vi "create_cache_directory_if_nonexistent.vi"(8 "error in (no error)":errorcluster, 10 "cache file":path, 11 "exists":bool) -> (0 "error out":errorcluster, 3 "cache file path":path)   [LabVIEW 2016]
uses:
  <userlib>/_OpenG.lib/file/file.llb/Strip Path - Traditional__ogtk.vi
  <userlib>/_OpenG.lib/file/file.llb/Build Path - Traditional__ogtk.vi
panel:
  out "created folders":bool
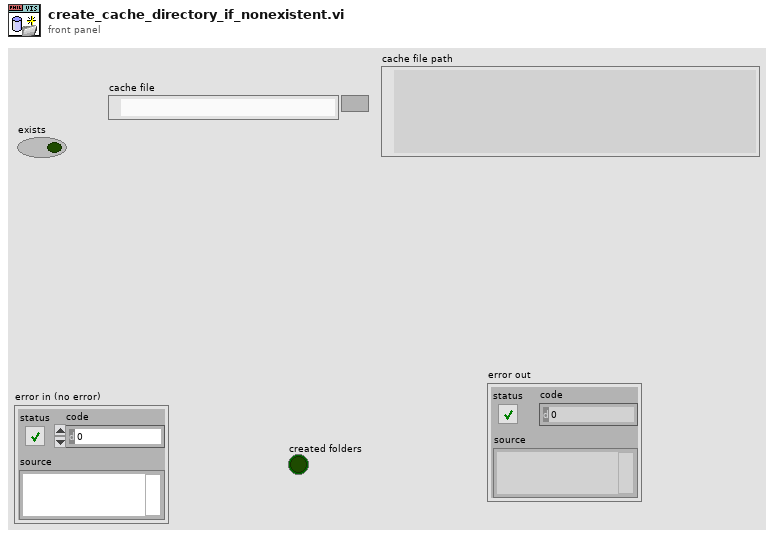
[diagram p1: front panel]
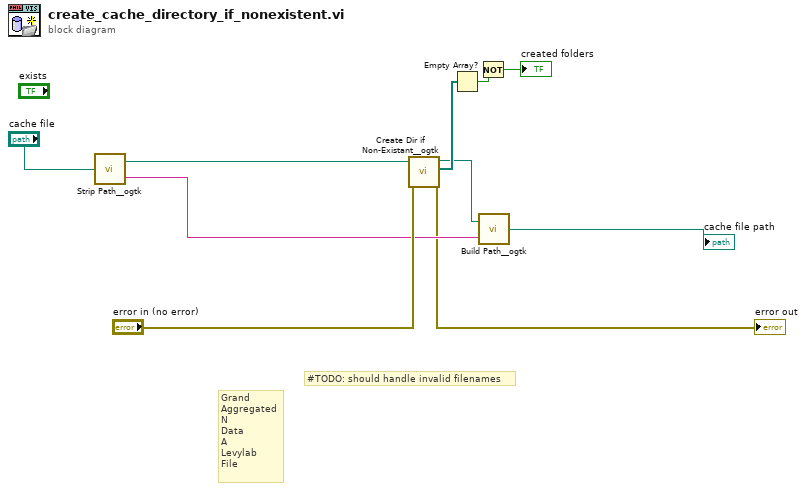
[diagram p0: block diagram]
diagram:
  # "Grand\nAggregated\nN\nData\nA\nLevylab\nFile"
  # "#TODO: should handle invalid filenames"
  n1 = call-poly <userlib>:"Strip Path__ogtk.vi"("path"="cache file") -> ("stripped path"=w4:path, "name"=w3:string)
  n2 = call <userlib>:"Create Dir if Non-Existant__ogtk.vi"("error in (no error)"="error in (no error)", "Directory Path"=w4) -> ("error out"=→"error out":errorcluster, "Created Directories"=w9:path[], "dup Directory Path"=w6:path)  [unwired: 7 in]
  n3 = Empty Array?(array=w9) -> (empty?=w8:bool)
  n4 = Not(x=w8) -> (.not. x?=→"created folders":bool)
  n5 = call-poly <userlib>:"Build Path__ogtk.vi"("name or relative path"=w3, "base path"=w6) -> ("appended path"=→"cache file path":path)
